vi "QE Reset N Chans.vi"(8 "Error In":errorcluster, 10 "QE Channels":u8[](array[numeric]), 11 "LINX Resource":T1) -> (0 "Error Out":errorcluster, 3 "LINX Resource":T1)   [LabVIEW 2013, in "LVH-LINX.lvlib"]
doc: "Set counter values to 0 for the specified quadrature encoder channels."
uses:
  LVH-LINX.lvlib
  Private/Type Defs/LINX Ref.ctl
  Private/Type Defs/Platform.ctl
  Private/Type Defs/Interface.ctl
  Private/Device/Type Defs/LINX Device Config.ctl
  Private/Device/Type Defs/TCP Config.ctl
  Private/Device/Type Defs/Channels.ctl
  Private/Type Defs/Peripheral.ctl
  Private/myRIO/myRIO.lvlib
  Private/Device/Device.lvlib
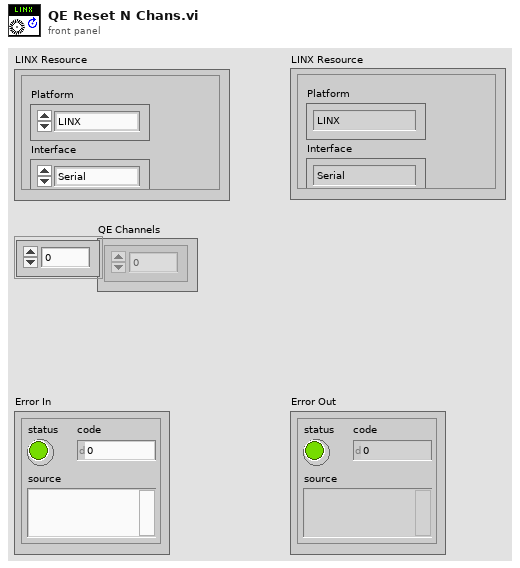
[diagram p1: front panel]
types:
  T1 = typedef "LVH-LINX.lvlib/LINX Ref.ctl" = cluster{"Platform":T2, "Interface":T3, "LINX Device Config":T4}
  T2 = typedef "LVH-LINX.lvlib/Platform.ctl" = enum16{"LINX", "myRIO"}
  T3 = typedef "LVH-LINX.lvlib/Interface.ctl" = enum16{"Serial", "TCP"}
  T4 = typedef "LVH-LINX.lvlib/Device.lvlib/LINX Device Config.ctl" = cluster{"Interface":T3, "COM Port":refnum<visa-resource-name>, "TCP Configuration":T5, "Device Family":u8, "Device ID":u8, "Device Name":string, "TCP Ref":refnum<k5>, "Channels":T6}
  T5 = typedef "LVH-LINX.lvlib/Device.lvlib/TCP Config.ctl" = cluster{"IP Address":string, "Port":u16}
  T6 = typedef "LVH-LINX.lvlib/Channels.ctl" = cluster{"DI Channels":u8[], "DO Channels":u8[], "AI":u8[], "AO":u8[], "PWM":u8[], "QE":u8[], "UART":u8[], "I2C 2":u8[], "SPI":u8[], "CAN":u8[], "AI Ref (V)":dbl, "AO Resolution (Bits)":u8, "AO Ref (V)":dbl}
  T7 = typedef "LVH-LINX.lvlib/Peripheral.ctl" = enum8{"DI", "DO", "AI", "AO", "PWM", "QE", "UART", "I2C", "SPI", "CAN"}
  T8 = typedef "DIO.lvlib/DIO Reference.ctl" = cluster{"myRIO Reference":T9, "DIO Channels List":T13}
  T9 = typedef "myRIO Generic Hardware Reference.ctl" = cluster{"myRIO Model":T10, "myRIO Hardware Reference":T11}
  T10 = typedef "Hardware Version Enum.ctl" = enum16{"Unknown", "myRIO-1900", "myRIO-1950"}
  T11 = typedef "myRIO v1.0 Reference.ctl" = cluster{"Generic FPGA Reference":T12, "Allow multiple opens":bool}
  T12 = typedef "Generic FPGA Reference.ctl" = refnum<k20>
  T13 = typedef "DIO Channels List.ctl" = T14[]
  T14 = typedef "DIO Channels Enum.ctl" = enum16{"Not Connected", "C/DIO0", "C/DIO1", "C/DIO2", "C/DIO3", "C/DIO4", "C/DIO5", "C/DIO6", "C/DIO7", "A/DIO0", "A/DIO1", "A/DIO2", "A/DIO3", "A/DIO4", "A/DIO5", "A/DIO6", "A/DIO7", "A/DIO8", "A/DIO9", "A/DIO10", "A/DIO11", "A/DIO12", "A/DIO13", "A/DIO14", "A/DIO15", "B/DIO0", "B/DIO1", "B/DIO2", "B/DIO3", "B/DIO4", "B/DIO5", "B/DIO6", "B/DIO7", "B/DIO8", "B/DIO9", "B/DIO10", "B/DIO11", "B/DIO12", "B/DIO13", "B/DIO14", "B/DIO15", "LED0", "LED1", "LED2", "LED3", "Button0"}
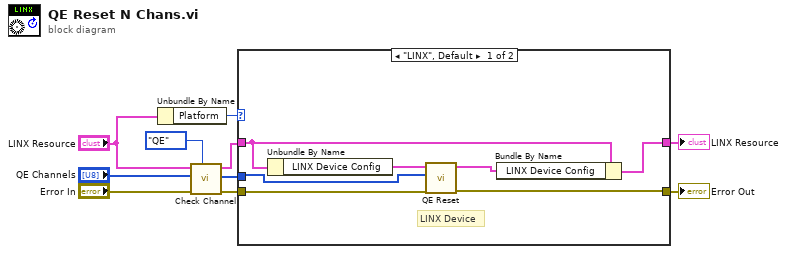
[diagram p0: block diagram]
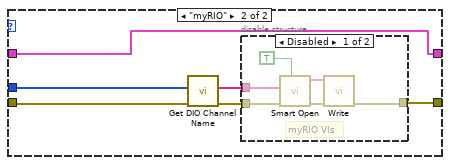
[diagram p2: hidden frame]
diagram:
  n1 = Unbundle By Name("LINX Resource") -> ("Platform"=w10:T2)
  n2 = call "Check Channel.vi"("Peripheral"=Peripheral."QE", "Error In"="Error In", "Channels"="QE Channels", "LINX Resource"="LINX Resource") -> ("Error Out"=w3:errorcluster, "Channels"=w2:u8[], "LINX Resource"=w5:T1)  [unwired: 5 in]
  n3 = case shown="\"LINX\", Default" w10 {
    tunnel: w3 -> [w13 w22]
    tunnel: w5 -> [w17 w23]
    tunnel: [w12 w19] -> w9
    tunnel: [w16 w23] -> w8
    tunnel: w2 -> [w14 w18]
    frame "LINX", Default {
      # "LINX Device"
      n4 = Unbundle By Name(w17) -> ("LINX Device Config"=w15:T4)
      n5 = call "QE Reset.vi"("Error In"=w13, "QE Channels"=w14, "LINX Device Config"=w15) -> ("Error Out"=w12:errorcluster, "LINX Device Config"=w11:T4)  [unwired: 7 in]
      n6 = Bundle By Name(cluster=w17, "LINX Device Config"=w11) -> (w16:T1)
    }
    frame "myRIO" {
      n7 = call "Get DIO Channel Name.vi"("Error In"=w22, "DIO Channel Nums"=w18) -> ("Error Out"=w20:errorcluster, "DIO Channels"=w21:string[])  [unwired: 8 in]
      n8 = disable-structure shown="Disabled" {
        disable-tunnel: w21 -> [w26 _]
        disable-tunnel: w20 -> [w27 w30]
        disable-tunnel: [w29 w30] -> w19
        frame Disabled {
          # "myRIO VIs"
          n9 = call <vilib>:"Smart Open.vi"("Allow multiple opens?"=TRUE, "error in (no error)"=w27, "Channel Names"=w26) -> ("error out"=w28:errorcluster, "DIO Ref Out"=w25:T8)  [unwired: 7 in]
          n10 = call <vilib>:"Write.vi"("error in (no error)"=w28, "DIO Ref In"=w25) -> ("error out"=w29:errorcluster)  [unwired: 7 in, 1 out]
        }
        frame Enabled {
          # "myRIO Support Disabled"
        }
      }
    }
  }
  "Error Out" <- w9
  "LINX Resource" <- w8
